vi "Node - Writer.vi"(8 "error in (no error)":errorcluster, 9 "Writing Segment":T1, 10 "PXImc Writing Session In":refnum<k21>, 11 "Master Table Ref In":refnum<data-value>) -> (0 "error out":errorcluster)   [LabVIEW 2016, in "PXImc Router.lvlib"]
uses:
  PXImc Router.lvlib
  Controls/Table Index-Size.ctl
  <vilib>/pximc/Acquire Write Region (DBL).vi
  <vilib>/pximc/nipximc.lvlib
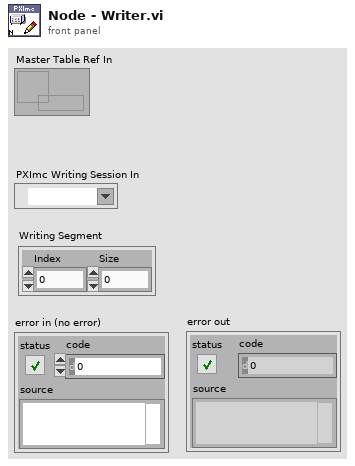
[diagram p1: front panel]
types:
  T1 = typedef "PXImc Router.lvlib/Table Index-Size.ctl" = cluster{"Index":u32, "Size":u32}
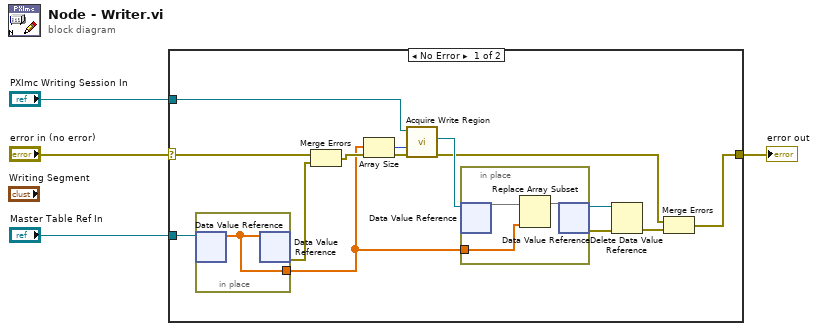
[diagram p0: block diagram]
diagram:
  n1 = case shown="No Error" "error in (no error)" {
    selector: "error in (no error)" -> [w14 w22]
    tunnel: "PXImc Writing Session In" -> [w17 _]
    tunnel: "Master Table Ref In" -> [w16 _]
    tunnel: [w15 w22] -> w3
    frame No Error {
      n2 = in-place {
        in-place-border: [w21] -> w5
        n3 = in-place-dvr #1(w16) -> (w21:dbl[])  [unwired: 1 out]
        n4 = in-place-dvr #1(w21) -> (w7:errorcluster)  [unwired: 1 out]
      }
      n5 = Merge Errors(w14, w7) -> (w6:errorcluster)
      n6 = Array Size(array=w5) -> (size(s)=w8:i32)
      n7 = call-poly <vilib>:"Acquire Write Region.vi"("error in (no error)"=w6, "number of elements"=w8, "session in"=w17) -> ("error out"=w9:errorcluster, "write region reference"=w10:refnum<data-value>)  [unwired: 5 in, 2 out]
      n8 = in-place {
        in-place-border: w5 -> [w18]
        n9 = in-place-dvr #2(w10) -> (w20:dbl[])  [unwired: 1 out]
        n10 = Replace Array Subset(array=w20, new element=w18) -> (w19:dbl[])  [unwired: 1 in]
        n11 = in-place-dvr #2(w19) -> (w11:refnum<data-value>, w13:errorcluster)
      }
      n12 = Delete Data Value Reference(data value reference=w11, error in=w13) -> (error out=w12:errorcluster)  [unwired: 1 out]
      n13 = Merge Errors(w9, w12) -> (w15:errorcluster)
    }
    frame Error {
    }
  }
  "error out" <- w3
